vi "KalmanFilter_GetK.vi"(11 "in KalmanFilter":T2) -> (3 "K":T1)   [LabVIEW 2019, in "Trajectory_Library.lvlib"]
doc: "Returns the steady-state Kalman gain matrix K.\n \nInputs:\n - KalmanFilter -- filter data cluster\n\nOutputs:\n - K - The steady-state Kalman gain matrix K."
uses:
  Trajectory_Library.lvlib
  TypeDef/KALMAN_FILTER.ctl
  <vilib>/Analysis/Matrix/Datatypes/RealMatrix.ctl
  TypeDef/LINEAR_SYSTEM.ctl
  <vilib>/Analysis/Matrix/NI_Matrix.lvlib
panel:
  # "Steady State Gain  \n<States,Outputs>"
  # "State Estimate <Statess,1>"
  # "<States,States>"
  # "<States,Inputs>"
  # "<Outputs,States>"
  # "<Outputs,Inputs>"
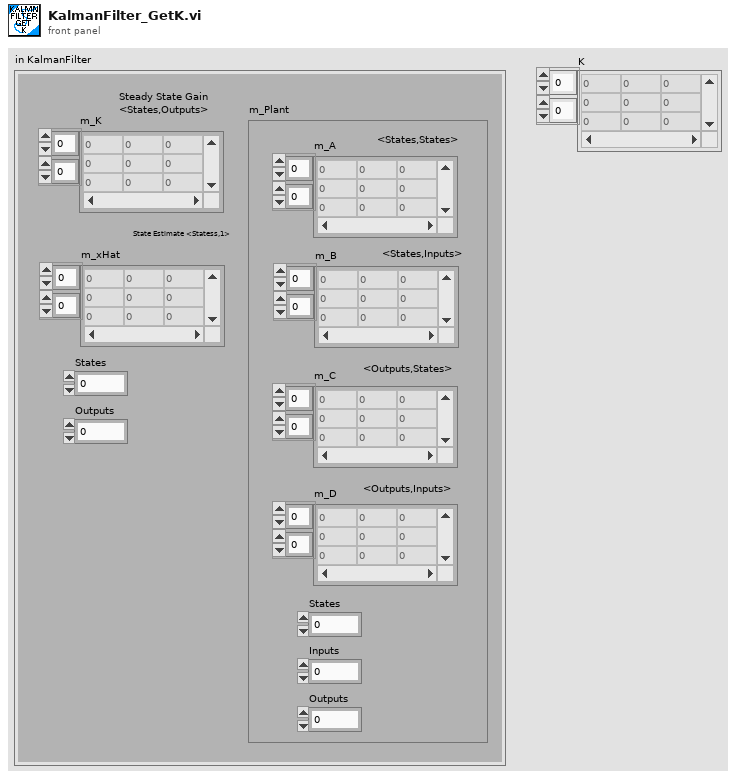
[diagram p1: front panel]
types:
  T1 = typedef "NI_Matrix.lvlib/RealMatrix.ctl" = dbl[][]
  T2 = typedef "Trajectory_Library.lvlib/KALMAN_FILTER.ctl" = cluster{"m_K":T1, "m_xHat":T1, "States":i32, "Outputs":i32, "m_Plant":T3}
  T3 = typedef "Trajectory_Library.lvlib/LINEAR_SYSTEM.ctl" = cluster{"m_A":T1, "m_B":T1, "m_C":T1, "m_D":T1, "States":i32, "Inputs":i32, "Outputs":i32}
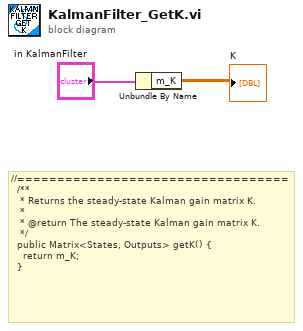
[diagram p0: block diagram]
diagram:
  # "//==================================\n  /**\n   * Returns the steady-state Kalman gain matrix K.\n   *\n   * @return The steady-state Kalman gain matrix K.\n   */\n  public Matrix<States, Outputs> getK() {\n    return m_K;\n  }"
  n1 = Unbundle By Name("in KalmanFilter") -> ("m_K"=→"K":T1)
